vi "BCU诊断标定.vi"(8 "CAN端口":u16(ring), 9 "设备索引号":u16(ring), 10 "CAN卡类型":u32(ring)=21, 11 "Myindex":dbl=1.0) -> (3 "成功":bool)   [LabVIEW 2013] (continued)
              n483 = property class="Tree (严格)"(reference=w821, "Active Item Row Number"=9 ("活动项:行数"), "Disabled?"=w795, "Active Item Row Number"=1 ("活动项:行数"), "Disabled?"=w794, "Active Item Row Number"=0 ("活动项:行数"), "Disabled?"=w799, "Active Item Row Number"=3 ("活动项:行数"), "Disabled?"=w813, "Active Item Row Number"=4 ("活动项:行数"), "Disabled?"=w812, "Active Item Row Number"=5 ("活动项:行数"), "Disabled?"=w811, "Active Item Row Number"=6 ("活动项:行数"), "Disabled?"=w810, "Active Item Row Number"=7 ("活动项:行数"), "Disabled?"=w809, "Active Item Row Number"=8 ("活动项:行数"), "Disabled?"=w808, "Active Item Row Number"=11 ("活动项:行数"), "Disabled?"=w807, "Active Item Row Number"=12 ("活动项:行数"), "Disabled?"=w806, "Active Item Row Number"=13 ("活动项:行数"), "Disabled?"=w805, "Active Item Row Number"=2 ("活动项:行数"), "Disabled?"=w804, "Active Item Row Number"=10 ("活动项:行数"), "Disabled?"=w803, "Active Item Row Number"=14 ("活动项:行数"), "Disabled?"=w802) -> ()  [unwired: 1 in, 2 out]
            }
            frame #2 {
              w864 = 18
              # "一二三级故障"
              n484 = global read "功能码全局.vi" "主板故障阀值9"() -> (w870:bool[])
              n485 = Index Array(array=w870) -> (element #3=w869:bool, element #4=w866:bool, element #5=w863:bool, element #6=w868:bool, element #7=w865:bool, element #8=w862:bool)  [unwired: 8 in, 2 out]
              n486 = Not Or(1:w868, 2:w869) -> (0:w858:bool)
              n487 = Not Or(1:w865, 2:w866) -> (0:w856:bool)
              n488 = Not Or(1:w862, 2:w863) -> (0:w857:bool)
              n489 = for {
                N: w864 -> [_]
                tunnel: w859 -> [w890]
                tunnel: w858 -> [w886]
                tunnel: [w885] -> w867
                i -> [w888]
                n490 = Add(x=w888, y=15) -> (x+y=w889:i32)
                n491 = property class="Tree (严格)"(reference=w890, "Active Item Row Number"=w889, "Disabled?"=w886) -> (error out=w885:errorcluster)  [unwired: 1 in, 1 out]
              }
              n492 = for {
                N: w864 -> [_]
                tunnel: w859 -> [w884]
                tunnel: w856 -> [w880]
                tunnel: w867 -> [w879]
                tunnel: [w878] -> w861
                i -> [w882]
                n493 = Add(x=w882, y=33) -> (x+y=w883:i32)
                n494 = property class="Tree (严格)"(reference=w884, error in=w879, "Active Item Row Number"=w883, "Disabled?"=w880) -> (error out=w878:errorcluster)  [unwired: 1 out]
              }
              n495 = for {
                N: w864 -> [_]
                tunnel: w859 -> [w877]
                tunnel: w857 -> [w873]
                tunnel: w861 -> [w872]
                tunnel: [w871] -> w860
                i -> [w875]
                n496 = Add(x=w875, y=51) -> (x+y=w876:i32)
                n497 = property class="Tree (严格)"(reference=w877, error in=w872, "Active Item Row Number"=w876, "Disabled?"=w873) -> (error out=w871:errorcluster)  [unwired: 1 out]
              }
              n498 = call <vilib>:"Clear Errors.vi"("error in (no error)"=w860) -> ()  [unwired: 6 in, 1 out]
            }
          }
        }
        frame Enabled {
        }
      }
      n499 = disable-structure shown="禁用" {
        disable-tunnel: [w543 _] -> w542
        frame Disabled {
          n500 = control-ref of="从板选项"() -> (w544:refnum<vi>)
          n501 = stacked-sequence {
            tunnel: w544 -> [w547 w584 w626]
            tunnel: [w545 _ _] -> w543
            frame #0 {
              n502 = global read "功能码全局.vi" "15"() -> (w570:bool[])
              n503 = global read "功能码全局.vi" "16"() -> (w561:bool[])
              n504 = Index Array(array=w570) -> (element #1=w569:bool, element #2=w567:bool, element #3=w565:bool, element #4=w563:bool, element #5=w568:bool, element #6=w566:bool, element #7=w564:bool, element #8=w562:bool)  [unwired: 8 in]
              n505 = Index Array(array=w561) -> (element #5=w552:bool, element #6=w560:bool, element #7=w551:bool, element #8=w559:bool)  [unwired: 8 in, 4 out]
              n506 = Not Or(1:w559, 2:w560) -> (0:w549:bool)
              n507 = Not Or(1:w551, 2:w552) -> (0:w550:bool)
              n508 = Not Or(1:w568, 2:w569) -> (0:w555:bool)
              n509 = Not Or(1:w566, 2:w567) -> (0:w556:bool)
              n510 = Not Or(1:w564, 2:w565) -> (0:w557:bool)
              n511 = Not Or(1:w562, 2:w563) -> (0:w558:bool)
              n512 = Compound Arithmetic op=OR(w555, w556, w557, w558, w549) -> (w554:bool)
              "从板项目信息" <- w554
              n513 = property class="Tree (严格)"(reference=w547, "Active Item Row Number"=1 ("活动项:行数"), "Disabled?"=w554, "Active Item Row Number"=2 ("活动项:行数"), "Disabled?"=w555, "Active Item Row Number"=3 ("活动项:行数"), "Disabled?"=w556, "Active Item Row Number"=4 ("活动项:行数"), "Disabled?"=w557, "Active Item Row Number"=5 ("活动项:行数"), "Disabled?"=w558, "Active Item Row Number"=0 ("活动项:行数"), "Disabled?"=w550) -> (error out=w546:errorcluster)  [unwired: 1 in, 1 out]
              n514 = for {
                N: 8 -> [_]
                tunnel: w547 -> [w582]
                tunnel: w549 -> [w578]
                tunnel: w546 -> [w577]
                tunnel: [w576] -> w545
                i -> [w580]
                n515 = Add(x=w580, y=6) -> (x+y=w581:i32)
                n516 = property class="Tree (严格)"(reference=w582, error in=w577, "Active Item Row Number"=w581, "Disabled?"=w578) -> (error out=w576:errorcluster)  [unwired: 1 out]
              }
              n517 = call <vilib>:"Clear Errors.vi"("error in (no error)"=w545) -> ()  [unwired: 6 in, 1 out]
            }
            frame #1 {
              w595 = 8
              n518 = global read "功能码全局.vi" "18"() -> (w604:bool[])
              n519 = Index Array(array=w604) -> (element #1=w587:bool, element #2=w588:bool, element #3=w603:bool, element #4=w598:bool, element #5=w592:bool, element #6=w602:bool, element #7=w597:bool, element #8=w591:bool)  [unwired: 8 in]
              n520 = Not Or(1:w588, 2:w587) -> (0:w583:bool)
              n521 = property class="Tree (严格)"(reference=w584, "Active Item Row Number"=46 ("活动项:行数"), "Disabled?"=w583, "Active Item Row Number"=47 ("活动项:行数"), "Disabled?"=w583, "Active Item Row Number"=48 ("活动项:行数"), "Disabled?"=w583) -> ()  [unwired: 1 in, 2 out]
              n522 = Not Or(1:w591, 2:w592) -> (0:w590:bool)
              n523 = Not Or(1:w602, 2:w603) -> (0:w601:bool)
              n524 = Not Or(1:w597, 2:w598) -> (0:w596:bool)
              n525 = for {
                N: w595 -> [_]
                tunnel: w584 -> [w625]
                tunnel: w601 -> [w621]
                tunnel: "error out" -> [w620]
                tunnel: [w619] -> w599
                i -> [w623]
                n526 = Add(x=w623, y=14) -> (x+y=w624:i32)
                n527 = property class="Tree (严格)"(reference=w625, error in=w620, "Active Item Row Number"=w624, "Disabled?"=w621) -> (error out=w619:errorcluster)  [unwired: 1 out]
              }
              n528 = for {
                N: w595 -> [_]
                tunnel: w584 -> [w618]
                tunnel: w596 -> [w614]
                tunnel: w599 -> [w613]
                tunnel: [w612] -> w594
                i -> [w616]
                n529 = Add(x=w616, y=22) -> (x+y=w617:i32)
                n530 = property class="Tree (严格)"(reference=w618, error in=w613, "Active Item Row Number"=w617, "Disabled?"=w614) -> (error out=w612:errorcluster)  [unwired: 1 out]
              }
              n531 = for {
                N: w595 -> [_]
                tunnel: w584 -> [w611]
                tunnel: w590 -> [w607]
                tunnel: w594 -> [w606]
                tunnel: [w605] -> w593
                i -> [w609]
                n532 = Add(x=w609, y=30) -> (x+y=w610:i32)
                n533 = property class="Tree (严格)"(reference=w611, error in=w606, "Active Item Row Number"=w610, "Disabled?"=w607) -> (error out=w605:errorcluster)  [unwired: 1 out]
              }
              n534 = call <vilib>:"Clear Errors.vi"("error in (no error)"=w593) -> ()  [unwired: 6 in, 1 out]
            }
            frame #2 {
              n535 = global read "功能码全局.vi" "23"() -> (w650:bool[])
              n536 = global read "功能码全局.vi" "24"() -> (w648:bool[])
              n537 = Index Array(array=w650) -> (element #3=w649:bool, element #4=w646:bool, element #5=w644:bool, element #6=w642:bool, element #7=w640:bool, element #8=w638:bool)  [unwired: 8 in, 2 out]
              n538 = Index Array(array=w648) -> (element #3=w647:bool, element #4=w645:bool, element #5=w643:bool, element #6=w641:bool, element #7=w639:bool, element #8=w637:bool)  [unwired: 8 in, 2 out]
              n539 = Not Or(1:w647, 2:w649) -> (0:w636:bool)
              n540 = Not Or(1:w645, 2:w646) -> (0:w631:bool)
              n541 = Not Or(1:w643, 2:w644) -> (0:w632:bool)
              n542 = Not Or(1:w641, 2:w642) -> (0:w633:bool)
              n543 = Not Or(1:w639, 2:w640) -> (0:w635:bool)
              n544 = Not Or(1:w637, 2:w638) -> (0:w634:bool)
              n545 = Build Array(w636, w636, w635, w634, w633, w632, w631) -> (w629:bool[])
              n546 = And Array Elements(Boolean array=w629) -> (logical AND=w630:bool)
              n547 = Insert Into Array(array=w629, index=0 ("索引"), new element=w630) -> (w627:bool[])
              n548 = for {
                N: 8 -> [_]
                tunnel: w626 -> [w660]
                tunnel: w627 -> [w656] mode=indexing
                tunnel: errorcluster {"status"=FALSE, "code"=0, "source"=""} ("error out 2") -> [w655]
                tunnel: [w654] -> w652
                i -> [w658]
                n549 = Add(x=w658, y=38) -> (x+y=w659:i32)
                n550 = property class="Tree (严格)"(reference=w660, error in=w655, "Active Item Row Number"=w659, "Disabled?"=w656) -> (error out=w654:errorcluster)  [unwired: 1 out]
              }
              n551 = call <vilib>:"Clear Errors.vi"("error in (no error)"=w652) -> ()  [unwired: 6 in, 1 out]
            }
          }
        }
        frame Enabled {
        }
      }
    }
  }
  n552 = Obtain Queue(name (unnamed)=w46, element data type=w46, error in (no error)=w34) -> (queue out=w45:refnum<queue>, error out=w8:errorcluster)  [unwired: 2 in, 1 out]
  n553 = Number To Decimal String(number="Myindex") -> (decimal integer string=w2:string)  [unwired: 1 in]
  n554 = Obtain Queue(name (unnamed)=w2, element data type="读参数") -> (queue out=w39:refnum<queue>, error out=w38:errorcluster)  [unwired: 3 in, 1 out]
  n555 = call <vilib>:"Open Config Data.vi"("error in (no error)"=w8, "configuration file path"=path "D:/BlueWay/BMU从板号.ini") -> ("error out"=w6:errorcluster, "refnum"=w7:T19)  [unwired: 7 in, 1 out]
  n556 = call-poly <vilib>:"Read Key.vi"("section"=w11, "error in (no error)"=w6, "default value"="BNET0001", "key"=w11, "refnum"=w7) -> ("error out"=w12:errorcluster, "value"=w4:string, "refnum out"=w13:T19)  [unwired: 3 in, 1 out]
  n557 = disable-structure shown="启用" {
    disable-tunnel: w45 -> [w898 _]
    disable-tunnel: w8 -> [w897 _]
    disable-tunnel: w37 -> [w892 _]
    disable-tunnel: w34 -> [w891 _]
    frame Enabled {
      n558 = while {
        tunnel: w898 -> [w907]
        tunnel: w897 -> [w906]
        tunnel: [w905] -> w896
        tunnel: [w904] -> w895
        tunnel: w892 -> [_]
        tunnel: w891 -> [_]
        stop <- w903 stop-if-true
        n559 = event shown="[2] 前面板关闭？" {
          selector: _ -> [_ _ _ _ _ _ _ _ _ _ _ _ _ _ _ _ _ _ _ _ _ _ _ _ _ _ _ _ _ _ _ _ _ _ _ _ _ _ _ _ _ _ _ _ _ _ _ _ _ _ _ _ _]
          dyn-events: _ -> [_ _ _ _ _ _ _ _ _ _ _ _ _ _ _ _ _ _ _ _ _ _ _ _ _ _ _ _ _ _ _ _ _ _ _ _ _ _ _ _ _ _ _ _ _ _ _ _ _ _ _ _ _]
          timeout: 200 -> [_ _ _ _ _ _ _ _ _ _ _ _ _ _ _ _ _ _ _ _ _ _ _ _ _ _ _ _ _ _ _ _ _ _ _ _ _ _ _ _ _ _ _ _ _ _ _ _ _ _ _ _ _]
          tunnel: [w908 w911 w951 _ _ _ _ _ _ _ _ _ _ _ _ _ _ _ _ _ _ _ _ _ _ _ _ _ _ _ _ _ _ _ _ _ _ _ _ _ _ _ _ _ _ _ _ _ _ _ _ _ _] -> w902
          tunnel: w907 -> [w910 w914 w950 _ w991 w1002 w1013 w1024 w1035 w1046 w1057 w1068 w1079 w1090 w1101 w1112 w1128 w1651 w2063 w2088 w2116 w2219 w2292 w2305 w2315 w2361 _ _ w2411 w2478 w2545 w2612 w2679 w2746 w2813 w2881 w2949 w3016 w3083 w3153 w3164 w3203 w3243 w3283 w3323 w3361 w3421 w3456 w3492 w3525 w3595 w3628 w3661]
          tunnel: w906 -> [w909 w913 w949 _ w990 w1001 w1012 w1023 w1034 w1045 w1056 w1067 w1078 w1089 w1100 w1111 w1127 w1650 w2062 w2087 w2115 w2218 w2290 w2303 w2314 w2360 _ _ w2410 w2477 w2544 w2611 w2678 w2745 w2812 w2880 w2948 w3015 w3082 w3151 w3163 w3202 w3242 w3282 w3322 w3360 w3420 w3455 w3491 w3524 w3594 w3627 w3660]
          tunnel: [w910 w914 w950 _ w991 w1002 w1013 w1024 w1035 w1046 w1057 w1068 w1079 w1090 w1101 w1112 w1128 w1651 w2063 w2088 w2116 w2219 w2291 w2304 w2315 w2361 _ _ w2411 w2478 w2545 w2612 w2679 w2746 w2813 w2881 w2949 w3016 w3083 w3152 w3162 w3201 w3241 w3281 w3321 w3361 w3419 w3454 w3490 w3523 w3593 w3626 w3659] -> w905
          tunnel: [w909 w913 w949 _ w990 w1001 w1012 w1023 w1034 w1045 w1056 w1067 w1078 w1089 w1100 w1111 w1127 w1650 w2062 w2087 w2115 w2218 w2289 w2302 w2314 w2360 _ _ w2410 w2477 w2544 w2611 w2678 w2745 w2812 w2880 w2948 w3015 w3082 w3150 w3161 w3200 w3240 w3280 w3320 w3360 w3418 w3453 w3489 w3522 w3592 w3625 w3658] -> w904
          tunnel: [_ _ _ _ _ _ _ _ _ _ _ _ _ _ _ _ _ _ _ _ _ _ _ _ _ _ _ _ _ _ _ _ _ _ _ _ _ _ _ _ w3161 w3200 w3240 w3280 w3320 _ w3418 w3453 w3489 w3522 w3592 w3625 w3658] -> w901
          event Timeout {
            n560 = event-data() -> ()  [unwired: 3 out]
            n561 = local read "停止"() -> (w908:bool)
          }
          event "停止": Value Change {
            n562 = event-data() -> ("NewVal"=w912:bool)  [unwired: 5 out]
            n563 = stacked-sequence {
              tunnel: w912 -> [w931 _]
              tunnel: [w931 _] -> w911
              frame #0 {
                n564 = global read "配置文件全局.vi" "诊断标定读取地址"() -> (w915:path)
                n565 = call <vilib>:"Application Directory.vi"() -> ("Application Directory"=w925:path)
                n566 = property class="VI"("FP.State"=T24."Hidden" ("前面板窗口:状态")) -> (reference out=w927:refnum<vi>, error out=w926:errorcluster)  [unwired: 2 in]
                n567 = Build Path(base path=w925, name or relative path="config.ini" ("名称或相对路径")) -> (appended path=w923:path)
                n568 = call <vilib>:"Open Config Data.vi"("configuration file path"=w923) -> ("error out"=w920:errorcluster, "refnum"=w922:T19)  [unwired: 8 in, 1 out]
                n569 = local write "停止"(TRUE ("停止")) -> ()
                n570 = property class="VI"(reference=w927, error in=w926, "Front Panel.Open"=FALSE ("前面板窗口:打开")) -> ()  [unwired: 2 out]
                n571 = call-poly <vilib>:"Write Key.vi"("section"="总信息", "error in (no error)"=w920, "value"=w915, "key"="诊断标定读取地址" ("section"), "refnum"=w922) -> ("error out"=w919:errorcluster, "refnum out"=w918:T19)  [unwired: 4 in, 1 out]
                n572 = call <vilib>:"Close Config Data.vi"("error in (no error)"=w919, "refnum"=w918) -> ("error out"=w917:errorcluster)  [unwired: 8 in, 1 out]
                n573 = call <vilib>:"Clear Errors.vi"("error in (no error)"=w917) -> ()  [unwired: 6 in, 1 out]
              }
              frame #1 {
                n574 = disable-structure shown="禁用" {
                  frame Disabled {
                    n575 = local read "设备索引号"() -> (w937:u16)
                    n576 = local read "CAN卡类型"() -> (w938:u32)
                    n577 = local read "CAN端口"() -> (w936:u16)
                    n578 = Build Array(7) -> (w933:i32[])
                    n579 = call "transmit-8.6.vi"("can卡类型"=w938, "设备索引号"=w937, "CAN端口"=w936, "ID"=418398080, "SendType"=u8 0, "Data"=w933) -> ()  [unwired: 3 in, 11 out]
                  }
                  frame Enabled {
                    w945 = u8 0 items=["Normal", "Listen Only"] ("工作方式")
                    w944 = u8 1 items=["Dual Filter", "Single Filter"] ("滤波方式")
                    n580 = local read "设备索引号"() -> (w940:u16)
                    n581 = local read "CAN卡类型"() -> (w939:u32)
                    n582 = local read "CAN端口"() -> (w941:u16)
                    n583 = call "CAN_Init-8.6.vi"("CAN卡类型"=w939, "设备索引号"=w940, "CAN端口"=w941, "操作类型"=enum16{"初始化CAN", "关闭CAN"}."初始化CAN", "滤波方式"=w944, "Accept Code"=u32 0, "簇"=T23 {"打开CAN"=FALSE, "初始化CAN"=TRUE, "开始CAN"=TRUE, "重启"=FALSE, "关闭CAN"=FALSE}, "Mask Code"=u32 4294967295 ("Accept Code"), "工作方式"=w945, "是否滤波"=FALSE) -> ()  [unwired: 4 in, 6 out]
                  }
                }
              }
            }
          }
          event Panel Close? {
            n584 = event-data() -> ()  [unwired: 5 out]
            n585 = stacked-sequence {
              tunnel: [w964 _] -> w951
              frame #0 {
                w964 = TRUE ("前面板窗口:打开")
                n586 = global read "配置文件全局.vi" "诊断标定读取地址"() -> (w953:path)
                n587 = call <vilib>:"Application Directory.vi"() -> ("Application Directory"=w963:path)
                n588 = property class="VI"("FP.State"=T24."Hidden" ("前面板窗口:状态")) -> (reference out=w966:refnum<vi>, error out=w965:errorcluster)  [unwired: 2 in]
                n589 = Build Path(base path=w963, name or relative path="config.ini" ("名称或相对路径")) -> (appended path=w961:path)
                n590 = call <vilib>:"Open Config Data.vi"("configuration file path"=w961) -> ("error out"=w958:errorcluster, "refnum"=w960:T19)  [unwired: 8 in, 1 out]
                n591 = property class="VI"(reference=w966, error in=w965, "Front Panel.Open"=FALSE ("前面板窗口:打开")) -> ()  [unwired: 2 out]
                n592 = call-poly <vilib>:"Write Key.vi"("section"="总信息", "error in (no error)"=w958, "value"=w953, "key"="诊断标定读取地址" ("section"), "refnum"=w960) -> ("error out"=w957:errorcluster, "refnum out"=w956:T19)  [unwired: 4 in, 1 out]
                n593 = call <vilib>:"Close Config Data.vi"("error in (no error)"=w957, "refnum"=w956) -> ("error out"=w955:errorcluster)  [unwired: 8 in, 1 out]
                n594 = call <vilib>:"Clear Errors.vi"("error in (no error)"=w955) -> ()  [unwired: 6 in, 1 out]
                n595 = local write "强制终止读写标记"(TRUE ("强制终止读写标记")) -> ()
                n596 = local write "停止"(w964) -> ()
              }
              frame #1 {
                w972 = u8 0 items=["Normal", "Listen Only"] ("工作方式")
                w973 = u8 1 items=["Dual Filter", "Single Filter"] ("滤波方式")
                n597 = local read "设备索引号"() -> (w977:u16)
                n598 = local read "CAN卡类型"() -> (w978:u32)
                n599 = local read "CAN端口"() -> (w976:u16)
                n600 = call "CAN_Init-8.6.vi"("CAN卡类型"=w978, "设备索引号"=w977, "CAN端口"=w976, "操作类型"=enum16{"初始化CAN", "关闭CAN"}."初始化CAN", "滤波方式"=w973, "Accept Code"=u32 0, "簇"=T23 {"打开CAN"=FALSE, "初始化CAN"=TRUE, "开始CAN"=TRUE, "重启"=FALSE, "关闭CAN"=FALSE}, "Mask Code"=u32 4294967295 ("Accept Code"), "工作方式"=w972, "是否滤波"=FALSE) -> ()  [unwired: 4 in, 6 out]
              }
            }
            n601 = event-data("Discard?"=w951) -> ()  [unwired: 1 in, 1 out]
          }
          event "终止读写按钮": Value Change {
            n602 = event-data() -> ("NewVal"=w979:bool)  [unwired: 6 out]
            n603 = case shown="真" w979 {
              frame False {
              }
              frame True {
                n604 = local write "强制终止读写标记"(TRUE ("强制终止读写标记")) -> ()
              }
            }
          }
          event "1": Value Change {
            w988 = FALSE ("1")
            n605 = event-data() -> ()  [unwired: 7 out]
            n606 = local write "主板2"(T8."项目信息" ("主从板")) -> ()
            n607 = Not(x=w988) -> (.not. x?=w987:bool)
            n608 = local write "1"(w987) -> ()
            n609 = local write "1 2"(w988) -> ()
            n610 = local write "1 3"(w988) -> ()
            n611 = local write "1 4"(w988) -> ()
            n612 = local write "1 5"(w988) -> ()
            n613 = local write "1 11"(w988) -> ()
            n614 = global read "功能码全局.vi" "主板监控2"() -> (w986:bool[])
            n615 = Index Array(array=w986, index=6 ("索引")) -> (element=w981:bool)
            n616 = Select(t=0, s=w981, f=1) -> (s? t:f=w982:i32)
            n617 = property on="项目信息" class="Tbl (严格)"("Disabled"=w982) -> ()  [unwired: 2 in, 2 out]
            n618 = property on="电池实际容量(A)" class="DigNum (严格)"("Disabled"=w982) -> ()  [unwired: 2 in, 2 out]
            n619 = property on="使用者" class="DigNum (严格)"("Disabled"=w982) -> ()  [unwired: 2 in, 2 out]
            n620 = property on="SOH(%)" class="DigNum (严格)"("Disabled"=w982) -> ()  [unwired: 2 in, 2 out]
            n621 = property on="电池额定容量(A)" class="DigNum (严格)"("Disabled"=w982) -> ()  [unwired: 2 in, 2 out]
            n622 = property on="SOC(%)" class="DigNum (严格)"("Disabled"=w982) -> ()  [unwired: 2 in, 2 out]
            n623 = property on="项目信息2" class="Clust (严格)"("DisabledEnum"=w982) -> ()  [unwired: 2 in, 2 out]
            n624 = property on="系统时钟" class="Str"("Disabled"=w982) -> ()  [unwired: 2 in, 2 out]
            n625 = property on="配置文件版本" class="Str"("Disabled"=w982) -> ()  [unwired: 2 in, 2 out]
            n626 = property on="车架(牌)号" class="Str"("Disabled"=w982) -> ()  [unwired: 2 in, 2 out]
            n627 = property on="产品编号" class="Str"("Disabled"=w982) -> ()  [unwired: 2 in, 2 out]
          }
          event "1 2": Value Change {
            w999 = FALSE ("1")
            n628 = event-data() -> ()  [unwired: 7 out]
            n629 = local write "主板2"(T8."一级故障阀值" ("主从板")) -> ()
            n630 = Not(x=w999) -> (.not. x?=w998:bool)
            n631 = local write "1"(w999) -> ()
            n632 = local write "1 2"(w998) -> ()
            n633 = local write "1 3"(w999) -> ()
            n634 = local write "1 4"(w999) -> ()
            n635 = local write "1 5"(w999) -> ()
            n636 = local write "1 11"(w999) -> ()
            n637 = global read "功能码全局.vi" "主板监控2"() -> (w997:bool[])
            n638 = Index Array(array=w997, index=6 ("索引")) -> (element=w992:bool)
            n639 = Select(t=0, s=w992, f=1) -> (s? t:f=w995:i32)
            n640 = property on="一级故障" class="Clust (严格)"("DisabledEnum"=w995) -> ()  [unwired: 2 in, 2 out]
          }
          event "1 3": Value Change {
            w1010 = FALSE ("1")
            n641 = event-data() -> ()  [unwired: 7 out]
            n642 = local write "主板2"(T8."二级故障阀值" ("主从板")) -> ()
            n643 = Not(x=w1010) -> (.not. x?=w1009:bool)
            n644 = local write "1"(w1010) -> ()
            n645 = local write "1 2"(w1010) -> ()
            n646 = local write "1 3"(w1009) -> ()
            n647 = local write "1 4"(w1010) -> ()
            n648 = local write "1 5"(w1010) -> ()
            n649 = local write "1 11"(w1010) -> ()
            n650 = global read "功能码全局.vi" "主板监控2"() -> (w1008:bool[])
            n651 = Index Array(array=w1008, index=6 ("索引")) -> (element=w1004:bool)
            n652 = Select(t=0, s=w1004, f=1) -> (s? t:f=w1003:i32)
            n653 = property on="一级故障 2" class="Clust (严格)"("DisabledEnum"=w1003) -> ()  [unwired: 2 in, 2 out]
          }
          event "1 4": Value Change {
            w1021 = FALSE ("1")
            n654 = event-data() -> ()  [unwired: 7 out]
            n655 = local write "主板2"(T8."三级故障阀值" ("主从板")) -> ()
            n656 = Not(x=w1021) -> (.not. x?=w1020:bool)
            n657 = local write "1"(w1021) -> ()
            n658 = local write "1 2"(w1021) -> ()
            n659 = local write "1 3"(w1021) -> ()
            n660 = local write "1 4"(w1020) -> ()
            n661 = local write "1 5"(w1021) -> ()
            n662 = local write "1 11"(w1021) -> ()
            n663 = global read "功能码全局.vi" "主板监控2"() -> (w1019:bool[])
            n664 = Index Array(array=w1019, index=6 ("索引")) -> (element=w1014:bool)
            n665 = Select(t=0, s=w1014, f=1) -> (s? t:f=w1017:i32)
            n666 = property on="一级故障 3" class="Clust (严格)"("DisabledEnum"=w1017) -> ()  [unwired: 2 in, 2 out]
          }
          event "1 5": Value Change {
            w1032 = FALSE ("1")
            n667 = event-data() -> ()  [unwired: 7 out]
            n668 = local write "主板2"(T8."控制参数" ("主从板")) -> ()
            n669 = Not(x=w1032) -> (.not. x?=w1031:bool)
            n670 = local write "1"(w1032) -> ()
            n671 = local write "1 2"(w1032) -> ()
            n672 = local write "1 3"(w1032) -> ()
            n673 = local write "1 4"(w1032) -> ()
            n674 = local write "1 5"(w1031) -> ()
            n675 = local write "1 11"(w1032) -> ()
            n676 = global read "功能码全局.vi" "主板监控2"() -> (w1028:bool[])
            n677 = Index Array(array=w1028, index=6 ("索引")) -> (element=w1026:bool)
            n678 = Select(t=0, s=w1026, f=1) -> (s? t:f=w1025:i32)
            n679 = property on="风机开启温度" class="DigNum (严格)"("Disabled"=w1025) -> ()  [unwired: 2 in, 2 out]
            n680 = property on="风机关闭温度" class="DigNum (严格)"("Disabled"=w1025) -> ()  [unwired: 2 in, 2 out]
            n681 = property on="加热开启温度" class="DigNum (严格)"("Disabled"=w1025) -> ()  [unwired: 2 in, 2 out]
            n682 = property on="加热关闭温度" class="DigNum (严格)"("Disabled"=w1025) -> ()  [unwired: 2 in, 2 out]
            n683 = property on="风机开启温差" class="DigNum (严格)"("Disabled"=w1025) -> ()  [unwired: 2 in, 2 out]
            n684 = property on="风机关闭温差" class="DigNum (严格)"("Disabled"=w1025) -> ()  [unwired: 2 in, 2 out]
            n685 = property on="加热控制参数" class="Clust (严格)"("DisabledEnum"=w1025) -> ()  [unwired: 2 in, 2 out]
            n686 = property on="最大允许总电压" class="DigNum (严格)"("Disabled"=w1025) -> ()  [unwired: 2 in, 2 out]
            n687 = property on="最大允许充电温度" class="DigNum (严格)"("Disabled"=w1025) -> ()  [unwired: 2 in, 2 out]
            n688 = property on="最小允许充电温度" class="DigNum (严格)"("Disabled"=w1025) -> ()  [unwired: 2 in, 2 out]
            n689 = property on="电流步长" class="DigNum (严格)"("Disabled"=w1025) -> ()  [unwired: 2 in, 2 out]
            n690 = property on="最大允许单体电压" class="DigNum (严格)"("Disabled"=w1025) -> ()  [unwired: 2 in, 2 out]
            n691 = property on="最小允许单体电压" class="DigNum (严格)"("Disabled"=w1025) -> ()  [unwired: 2 in, 2 out]
            n692 = property on="最大允许充电电流" class="DigNum (严格)"("Disabled"=w1025) -> ()  [unwired: 2 in, 2 out]
            n693 = property on="最小允许充电电流" class="DigNum (严格)"("Disabled"=w1025) -> ()  [unwired: 2 in, 2 out]
          }
          event "1 11": Value Change {
            w1043 = FALSE ("1")
            n694 = event-data() -> ()  [unwired: 7 out]
            n695 = local write "主板2"(T8."电池信息" ("主从板")) -> ()
            n696 = Not(x=w1043) -> (.not. x?=w1042:bool)
            n697 = local write "1"(w1043) -> ()
            n698 = local write "1 2"(w1043) -> ()
            n699 = local write "1 3"(w1043) -> ()
            n700 = local write "1 4"(w1043) -> ()
            n701 = local write "1 5"(w1043) -> ()
            n702 = local write "1 11"(w1042) -> ()
            n703 = global read "功能码全局.vi" "主板监控2"() -> (w1038:bool[])
            n704 = Index Array(array=w1038, index=6 ("索引")) -> (element=w1036:bool)
            n705 = Select(t=0, s=w1036, f=1) -> (s? t:f=w1039:i32)
            n706 = property on="电池串联" class="DigNum (严格)"("Disabled"=w1039) -> ()  [unwired: 2 in, 2 out]
            n707 = property on="电池并联" class="DigNum (严格)"("Disabled"=w1039) -> ()  [unwired: 2 in, 2 out]
            n708 = property on="电池包额定容量" class="DigNum (严格)"("Disabled"=w1039) -> ()  [unwired: 2 in, 2 out]
            n709 = property on="电池包额定能量(kWh)" class="DigNum (严格)"("Disabled"=w1039) -> ()  [unwired: 2 in, 2 out]
            n710 = property on="电池包额定总电压" class="DigNum (严格)"("Disabled"=w1039) -> ()  [unwired: 2 in, 2 out]
            n711 = property on="实际容量" class="DigNum (严格)"("Disabled"=w1039) -> ()  [unwired: 2 in, 2 out]
            n712 = property on="电池包组号" class="Str"("Disabled"=w1039) -> ()  [unwired: 2 in, 2 out]
            n713 = property on="电池生产日期" class="Str"("Disabled"=w1039) -> ()  [unwired: 2 in, 2 out]
            n714 = property on="电池厂家" class="Str"("Disabled"=w1039) -> ()  [unwired: 2 in, 2 out]
            n715 = property on="电池类型" class="Str"("Disabled"=w1039) -> ()  [unwired: 2 in, 2 out]
            n716 = property on="累计充电总安时" class="DigNum (严格)"("Disabled"=w1039) -> ()  [unwired: 2 in, 2 out]
            n717 = property on="累计放电总安时" class="DigNum (严格)"("Disabled"=w1039) -> ()  [unwired: 2 in, 2 out]
            n718 = property on="电池放空次数" class="DigNum (严格)"("Disabled"=w1039) -> ()  [unwired: 2 in, 2 out]
            n719 = property on="电池充满次数" class="DigNum (严格)"("Disabled"=w1039) -> ()  [unwired: 2 in, 2 out]
            n720 = property on="电池充电次数" class="DigNum (严格)"("Disabled"=w1039) -> ()  [unwired: 2 in, 2 out]
            n721 = property on="电池信息" class="Clust (严格)"("DisabledEnum"=w1039) -> ()  [unwired: 2 in, 2 out]
          }
          event "1 6": Value Change {
            w1054 = FALSE ("1 6")
            n722 = event-data() -> ()  [unwired: 7 out]
            n723 = local write "等级 2"(T21."从板信息" ("等级 2")) -> ()
            n724 = global read "功能码全局.vi" "主板监控2"() -> (w1049:bool[])
            n725 = Not(x=w1054) -> (.not. x?=w1053:bool)
            n726 = local write "1 6"(w1053) -> ()
            n727 = local write "1 7"(w1054) -> ()
            n728 = local write "1 8"(w1054) -> ()
            n729 = local write "1 9"(w1054) -> ()
            n730 = local write "1 10"(w1054) -> ()
            n731 = Index Array(array=w1049, index=6 ("索引")) -> (element=w1047:bool)
            n732 = Select(t=0, s=w1047, f=1) -> (s? t:f=w1050:i32)
            n733 = property on="项目信息 2" class="Tbl (严格)"("Disabled"=w1050) -> ()  [unwired: 2 in, 2 out]
            n734 = property on="加热控制参数" class="Clust (严格)"("Disabled"=w1050) -> ()  [unwired: 2 in, 2 out]
          }
          event "1 7": Value Change {
            w1065 = FALSE ("1 6")
            n735 = event-data() -> ()  [unwired: 7 out]
            n736 = global read "功能码全局.vi" "主板监控2"() -> (w1063:bool[])
            n737 = Index Array(array=w1063, index=6 ("索引")) -> (element=w1058:bool)
            n738 = local write "等级 2"(T21."一级故障阀值" ("等级 2")) -> ()
            n739 = Select(t=0, s=w1058, f=1) -> (s? t:f=w1059:i32)
            n740 = property on="一级故障 6" class="Clust (严格)"("DisabledEnum"=w1059) -> ()  [unwired: 2 in, 2 out]
            n741 = Not(x=w1065) -> (.not. x?=w1064:bool)
            n742 = local write "1 6"(w1065) -> ()
            n743 = local write "1 7"(w1064) -> ()
            n744 = local write "1 8"(w1065) -> ()
            n745 = local write "1 9"(w1065) -> ()
            n746 = local write "1 10"(w1065) -> ()
          }
          event "1 8": Value Change {
            w1076 = FALSE ("1 6")
            n747 = event-data() -> ()  [unwired: 7 out]
            n748 = global read "功能码全局.vi" "主板监控2"() -> (w1074:bool[])
            n749 = Index Array(array=w1074, index=6 ("索引")) -> (element=w1069:bool)
            n750 = local write "等级 2"(T21."二级故障阀值" ("等级 2")) -> ()
            n751 = Select(t=0, s=w1069, f=1) -> (s? t:f=w1070:i32)
            n752 = Not(x=w1076) -> (.not. x?=w1075:bool)
            n753 = property on="一级故障 7" class="Clust (严格)"("DisabledEnum"=w1070) -> ()  [unwired: 2 in, 2 out]
            n754 = local write "1 6"(w1076) -> ()
            n755 = local write "1 7"(w1076) -> ()
            n756 = local write "1 8"(w1075) -> ()
            n757 = local write "1 9"(w1076) -> ()
            n758 = local write "1 10"(w1076) -> ()
          }
          event "1 9": Value Change {
            w1087 = FALSE ("1 6")
            n759 = event-data() -> ()  [unwired: 7 out]
            n760 = global read "功能码全局.vi" "主板监控2"() -> (w1085:bool[])
            n761 = Index Array(array=w1085, index=6 ("索引")) -> (element=w1080:bool)
            n762 = Select(t=0, s=w1080, f=1) -> (s? t:f=w1081:i32)
            n763 = local write "等级 2"(T21."三级故障阀值" ("等级 2")) -> ()
            n764 = property on="一级故障 8" class="Clust (严格)"("DisabledEnum"=w1081) -> ()  [unwired: 2 in, 2 out]
            n765 = Not(x=w1087) -> (.not. x?=w1086:bool)
            n766 = local write "1 6"(w1087) -> ()
            n767 = local write "1 7"(w1087) -> ()
            n768 = local write "1 8"(w1087) -> ()
            n769 = local write "1 9"(w1086) -> ()
            n770 = local write "1 10"(w1087) -> ()
          }
          event "1 10": Value Change {
            w1098 = FALSE ("1 6")
            n771 = event-data() -> ()  [unwired: 7 out]
            n772 = global read "功能码全局.vi" "主板监控2"() -> (w1096:bool[])
            n773 = Index Array(array=w1096, index=6 ("索引")) -> (element=w1091:bool)
            n774 = Select(t=0, s=w1091, f=1) -> (s? t:f=w1092:i32)
            n775 = local write "等级 2"(T21."快换参数" ("等级 2")) -> ()
            n776 = property on="电池组信息" class="Clust (严格)"("Disabled"=w1092) -> ()  [unwired: 2 in, 2 out]
            n777 = Not(x=w1098) -> (.not. x?=w1097:bool)
            n778 = local write "1 6"(w1098) -> ()
            n779 = local write "1 7"(w1098) -> ()
            n780 = local write "1 8"(w1098) -> ()
            n781 = local write "1 9"(w1098) -> ()
            n782 = local write "1 10"(w1097) -> ()
          }
          event "1 12": Value Change {
            w1103 = FALSE ("1 6")
            n783 = event-data() -> ()  [unwired: 7 out]
            n784 = global read "功能码全局.vi" "主板监控2"() -> (w1110:bool[])
            n785 = Index Array(array=w1110, index=6 ("索引")) -> (element=w1106:bool)
            n786 = Select(t=0, s=w1106, f=1) -> (s? t:f=w1102:i32)
            n787 = local write "等级 2"(T14."均衡参数" ("等级 2")) -> ()
            n788 = property on="均衡参数" class="Clust (严格)"("DisabledEnum"=w1102) -> ()  [unwired: 2 in, 2 out]
            n789 = Not(x=w1103) -> (.not. x?=w1104:bool)
            n790 = local write "1 12"(w1104) -> ()
            n791 = local write "1 6"(w1103) -> ()
            n792 = local write "1 7"(w1103) -> ()
            n793 = local write "1 8"(w1103) -> ()
            n794 = local write "1 9"(w1103) -> ()
            n795 = local write "1 10"(w1103) -> ()
          }
          event "主板选项": Mouse Down {
            n796 = event-data() -> ("CtlRef"=w1126:refnum<vi>)  [unwired: 8 out]
            n797 = global read "功能码全局.vi" "主板监控2"() -> (w1115:bool[])
            n798 = property class="Tree (严格)"(reference=w1126) -> ("Value"=w1118:string)  [unwired: 1 in, 2 out]
            n799 = Index Array(array=w1115, index=6 ("索引")) -> (element=w1113:bool)
            n800 = case shown="\"温度个数\"" w1118 {
              tunnel: [T8."项目信息" ("主从板") T8."项目信息" ("主从板") T8."项目信息" ("主从板") T8."项目信息" ("主从板") T8."项目信息" ("主从板") T8."项目信息" ("主从板") T8."项目信息" ("主从板") T8."项目信息" ("主从板") T8."项目信息" ("主从板") T8."项目信息" ("主从板") T8."项目信息" ("主从板") T8."项目信息" ("主从板") T8."项目信息" ("主从板") T8."项目信息" ("主从板") T8."项目信息" ("主从板") T8."二级故障阀值" ("主从板") T8."三级故障阀值" ("主从板") T8."一级故障阀值" ("主从板") T8."控制参数" ("主从板") T8."控制参数" ("主从板") T8."电池信息" ("主从板") T8."电池信息" ("主从板") T8."电池信息" ("主从板") T8."电池信息" ("主从板") T8."电池信息" ("主从板") T8."项目信息" ("主从板")] -> w1125
              tunnel: [w1136 w1143 w1158 w1175 w1215 w1249 w1296 w1334 w1384 w1419 w1433 w1448 w1463 w1478 w1492 w1505 w1519 w1532 w1546 w1560 w1573 w1587 w1601 w1615 w1629 w1633] -> w1124
              tunnel: [w1137 w1144 w1159 w1176 w1216 w1250 w1297 w1335 w1385 w1420 w1434 w1449 w1464 w1479 w1493 w1505 w1519 w1531 w1546 w1560 w1573 w1587 w1601 w1615 w1629 w1634] -> w1123
              tunnel: [w1137 w1144 w1159 w1176 w1216 w1250 w1297 w1335 w1385 w1420 w1434 w1449 w1464 w1479 w1493 w1506 w1519 w1532 w1546 w1560 w1573 w1587 w1601 w1615 w1629 w1634] -> w1122
              tunnel: [w1137 w1144 w1159 w1176 w1216 w1250 w1297 w1335 w1385 w1420 w1434 w1449 w1464 w1479 w1493 w1505 w1518 w1532 w1546 w1560 w1573 w1587 w1601 w1615 w1629 w1634] -> w1121
              tunnel: [w1137 w1144 w1159 w1176 w1216 w1250 w1297 w1335 w1385 w1420 w1434 w1449 w1464 w1479 w1493 w1505 w1519 w1532 w1545 w1559 w1573 w1587 w1601 w1615 w1629 w1634] -> w1120
              tunnel: [w1137 w1144 w1159 w1176 w1216 w1250 w1297 w1335 w1385 w1420 w1434 w1449 w1464 w1479 w1493 w1505 w1519 w1532 w1546 w1560 w1572 w1586 w1600 w1614 w1628 w1634] -> w1119
              tunnel: [w1129 FALSE w1154 w1167 w1207 w1240 w1287 w1326 w1377 w1414 w1428 w1442 w1456 w1471 w1487 w1501 w1514 w1527 w1541 w1554 w1568 w1581 w1595 w1609 w1623 FALSE] -> w1117
              tunnel: [w1129 TRUE w1151 w1166 w1206 w1241 w1288 w1325 w1376 w1413 w1427 w1441 w1457 w1472 w1486 w1500 w1513 w1526 w1540 w1553 w1567 w1580 w1594 w1608 w1622 FALSE] -> w1116
              tunnel: w1113 -> [w1134 _ w1148 w1163 w1202 w1237 w1284 w1322 w1374 w1410 w1424 w1438 w1453 w1468 w1483 w1497 w1510 w1523 w1537 w1550 w1564 w1577 w1591 w1605 w1619 _]
              frame "项目信息" {
                w1137 = FALSE
                n801 = Select(t=0, s=w1134, f=1) -> (s? t:f=w1132:i32)
                n802 = property on="项目信息" class="Tbl (严格)"("Disabled"=w1132) -> ()  [unwired: 2 in, 2 out]
                n803 = property on="电池实际容量(A)" class="DigNum (严格)"("Disabled"=w1132) -> ()  [unwired: 2 in, 2 out]
                n804 = property on="使用者" class="DigNum (严格)"("Disabled"=w1132) -> ()  [unwired: 2 in, 2 out]
                n805 = property on="SOH(%)" class="DigNum (严格)"("Disabled"=w1132) -> ()  [unwired: 2 in, 2 out]
                n806 = property on="从板个数" class="DigNum (严格)"("NumText.BGColor"=u32 6618880) -> ()  [unwired: 2 in, 2 out]
                n807 = property on="电池额定容量(A)" class="DigNum (严格)"("Disabled"=w1132) -> ()  [unwired: 2 in, 2 out]
                n808 = property on="SOC(%)" class="DigNum (严格)"("Disabled"=w1132) -> ()  [unwired: 2 in, 2 out]
                n809 = property on="项目信息2" class="Clust (严格)"("DisabledEnum"=w1132) -> ()  [unwired: 2 in, 2 out]
                n810 = property on="系统时钟" class="Str"("Disabled"=w1132) -> ()  [unwired: 2 in, 2 out]
                n811 = property on="配置文件版本" class="Str"("Disabled"=w1132) -> ()  [unwired: 2 in, 2 out]
                n812 = property on="车架(牌)号" class="Str"("Disabled"=w1132) -> ()  [unwired: 2 in, 2 out]
                n813 = property on="产品编号" class="Str"("Disabled"=w1132) -> ()  [unwired: 2 in, 2 out]
                n814 = local read "项目信息结果"() -> (w1130:bool)
                n815 = Not(x=w1130) -> (.not. x?=w1129:bool)
                n816 = Not(x=w1137) -> (.not. x?=w1136:bool)
              }
              frame "校正时钟" {
                w1140 = 2
                w1144 = FALSE
                n817 = property on="从板个数" class="DigNum (严格)"("NumText.BGColor"=u32 13816530) -> ()  [unwired: 2 in, 2 out]
                n818 = property on="项目信息" class="Tbl (严格)"("Disabled"=w1140) -> ()  [unwired: 2 in, 2 out]
                n819 = property on="电池实际容量(A)" class="DigNum (严格)"("Disabled"=w1140) -> ()  [unwired: 2 in, 2 out]
                n820 = property on="使用者" class="DigNum (严格)"("Disabled"=w1140) -> ()  [unwired: 2 in, 2 out]
                n821 = property on="SOH(%)" class="DigNum (严格)"("Disabled"=w1140) -> ()  [unwired: 2 in, 2 out]
                n822 = property on="电池额定容量(A)" class="DigNum (严格)"("Disabled"=w1140) -> ()  [unwired: 2 in, 2 out]
                n823 = property on="SOC(%)" class="DigNum (严格)"("Disabled"=w1140) -> ()  [unwired: 2 in, 2 out]
                n824 = property on="系统时钟" class="Str"("Disabled"=w1140) -> ()  [unwired: 2 in, 2 out]
                n825 = property on="配置文件版本" class="Str"("Disabled"=w1140) -> ()  [unwired: 2 in, 2 out]
                n826 = property on="车架(牌)号" class="Str"("Disabled"=w1140) -> ()  [unwired: 2 in, 2 out]
                n827 = property on="项目信息2" class="Clust (严格)"("DisabledEnum"=w1140) -> ()  [unwired: 2 in, 2 out]
                n828 = property on="产品编号" class="Str"("Disabled"=w1140) -> ()  [unwired: 2 in, 2 out]
                n829 = Not(x=w1144) -> (.not. x?=w1143:bool)
              }
              frame "产品编号" {
                w1157 = 2
                w1159 = FALSE
                n830 = property on="项目信息" class="Tbl (严格)"("Disabled"=w1157) -> ()  [unwired: 2 in, 2 out]
                n831 = property on="电池实际容量(A)" class="DigNum (严格)"("Disabled"=w1157) -> ()  [unwired: 2 in, 2 out]
                n832 = property on="使用者" class="DigNum (严格)"("Disabled"=w1157) -> ()  [unwired: 2 in, 2 out]
                n833 = Select(t=0, s=w1148, f=1) -> (s? t:f=w1147:i32)
                n834 = property on="SOH(%)" class="DigNum (严格)"("Disabled"=w1157) -> ()  [unwired: 2 in, 2 out]
                n835 = property on="电池额定容量(A)" class="DigNum (严格)"("Disabled"=w1157) -> ()  [unwired: 2 in, 2 out]
                n836 = property on="SOC(%)" class="DigNum (严格)"("Disabled"=w1157) -> ()  [unwired: 2 in, 2 out]
                n837 = property on="产品编号" class="Str"("Disabled"=w1147) -> ()  [unwired: 2 in, 2 out]
                n838 = property on="项目信息2" class="Clust (严格)"("DisabledEnum"=w1147) -> ()  [unwired: 2 in, 2 out]
                n839 = property on="系统时钟" class="Str"("Disabled"=w1157) -> ()  [unwired: 2 in, 2 out]
                n840 = property on="配置文件版本" class="Str"("Disabled"=w1157) -> ()  [unwired: 2 in, 2 out]
                n841 = property on="车架(牌)号" class="Str"("Disabled"=w1157) -> ()  [unwired: 2 in, 2 out]
                n842 = property on="从板个数" class="DigNum (严格)"("NumText.BGColor"=u32 13816530) -> ()  [unwired: 2 in, 2 out]
                n843 = global read "功能码全局.vi" "主板项目信息5"() -> (w1155:bool[])
                n844 = global read "功能码全局.vi" "主板项目信息6"() -> (w1152:bool[])
                n845 = Index Array(array=w1155, index=0 ("索引")) -> (element=w1154:bool)
                n846 = Index Array(array=w1152, index=1 ("索引")) -> (element=w1151:bool)
                n847 = Not(x=w1159) -> (.not. x?=w1158:bool)
              }
              frame "电压个数" {
                w1174 = 2
                w1176 = FALSE
                n848 = local read "从板个数"() -> (w1173:dbl)
                n849 = property on="从板个数" class="DigNum (严格)"("NumText.BGColor"=u32 6618880) -> ()  [unwired: 2 in, 2 out]
                n850 = property on="电池实际容量(A)" class="DigNum (严格)"("Disabled"=w1174) -> ()  [unwired: 2 in, 2 out]
                n851 = property on="使用者" class="DigNum (严格)"("Disabled"=w1174) -> ()  [unwired: 2 in, 2 out]
                n852 = property on="SOH(%)" class="DigNum (严格)"("Disabled"=w1174) -> ()  [unwired: 2 in, 2 out]
                n853 = property on="电池额定容量(A)" class="DigNum (严格)"("Disabled"=w1174) -> ()  [unwired: 2 in, 2 out]
                n854 = property on="SOC(%)" class="DigNum (严格)"("Disabled"=w1174) -> ()  [unwired: 2 in, 2 out]
                n855 = property on="系统时钟" class="Str"("Disabled"=w1174) -> ()  [unwired: 2 in, 2 out]
                n856 = property on="配置文件版本" class="Str"("Disabled"=w1174) -> ()  [unwired: 2 in, 2 out]
                n857 = property on="车架(牌)号" class="Str"("Disabled"=w1174) -> ()  [unwired: 2 in, 2 out]
                n858 = property on="产品编号" class="Str"("Disabled"=w1174) -> ()  [unwired: 2 in, 2 out]
                n859 = Select(t=0, s=w1163, f=1) -> (s? t:f=w1162:i32)
                n860 = control-ref of="项目信息"() -> (w1172:refnum<vi>)
                n861 = stacked-sequence {
                  tunnel: w1173 -> [_ w1183 w1193]
                  tunnel: w1172 -> [w1178 w1182 w1194]
                  frame #0 {
                    w1179 = 0
                    n862 = Bundle(w1179, w1179) -> (w1181:cluster{i32, i32})  [unwired: 1 out]
                    n863 = property class="Tbl (严格)"(reference=w1178, "Index Values"=w1181) -> (error out=w1180:errorcluster)  [unwired: 1 in, 1 out]
                    n864 = call <vilib>:"Clear Errors.vi"("error in (no error)"=w1180) -> ()  [unwired: 7 out]
                  }
                  frame #1 {
                    n865 = for {
                      N: 10 -> [_]
                      tunnel: w1182 -> [w1192]
                      tunnel: w1183 -> [w1187]
                      i -> [w1186]
                      n866 = Compound Arithmetic op=ADD(0.0 ("值"), w1187, w1186) -> (w1189:dbl)
                      n867 = Bundle(w1189, 0) -> (w1191:cluster{dbl, i32})  [unwired: 1 out]
                      n868 = property class="Tbl (严格)"(reference=w1192, "Active Cell"=w1191, "Cell BG Color"=u32 16448250) -> ()  [unwired: 1 in, 2 out]
                    }
                  }
                  frame #2 {
                    n869 = for {
                      N: w1193 -> [_]
                      tunnel: w1194 -> [w1195]
                      i -> [w1196]
                      n870 = Bundle(w1196, 0) -> (w1200:cluster{i32, i32})  [unwired: 1 out]
                      n871 = property class="Tbl (严格)"(reference=w1195, "Active Cell"=w1200, "Cell BG Color"=u32 6618880) -> (error out=w1197:errorcluster)  [unwired: 1 in, 1 out]
                      n872 = call <vilib>:"Clear Errors.vi"("error in (no error)"=w1197) -> ()  [unwired: 7 out]
                    }
                  }
                }
                n873 = property on="项目信息" class="Tbl (严格)"("Disabled"=w1162) -> ()  [unwired: 2 in, 2 out]
                n874 = global read "功能码全局.vi" "主板项目信息5"() -> (w1170:bool[])
                n875 = global read "功能码全局.vi" "主板项目信息6"() -> (w1168:bool[])
                n876 = Index Array(array=w1170, index=1 ("索引")) -> (element=w1167:bool)
                n877 = Index Array(array=w1168, index=2 ("索引")) -> (element=w1166:bool)
                n878 = Not(x=w1176) -> (.not. x?=w1175:bool)
              }
              frame "通道电压数" {
                w1214 = 2
                w1216 = FALSE
                n879 = property on="从板个数" class="DigNum (严格)"("NumText.BGColor"=u32 13816530) -> ()  [unwired: 2 in, 2 out]
                n880 = property on="电池实际容量(A)" class="DigNum (严格)"("Disabled"=w1214) -> ()  [unwired: 2 in, 2 out]
                n881 = property on="使用者" class="DigNum (严格)"("Disabled"=w1214) -> ()  [unwired: 2 in, 2 out]
                n882 = property on="SOH(%)" class="DigNum (严格)"("Disabled"=w1214) -> ()  [unwired: 2 in, 2 out]
                n883 = property on="电池额定容量(A)" class="DigNum (严格)"("Disabled"=w1214) -> ()  [unwired: 2 in, 2 out]
                n884 = property on="SOC(%)" class="DigNum (严格)"("Disabled"=w1214) -> ()  [unwired: 2 in, 2 out]
                n885 = local read "从板个数"() -> (w1212:dbl)
                n886 = property on="系统时钟" class="Str"("Disabled"=w1214) -> ()  [unwired: 2 in, 2 out]
                n887 = property on="配置文件版本" class="Str"("Disabled"=w1214) -> ()  [unwired: 2 in, 2 out]
                n888 = property on="车架(牌)号" class="Str"("Disabled"=w1214) -> ()  [unwired: 2 in, 2 out]
                n889 = property on="产品编号" class="Str"("Disabled"=w1214) -> ()  [unwired: 2 in, 2 out]
                n890 = control-ref of="项目信息"() -> (w1213:refnum<vi>)
                n891 = stacked-sequence {
                  tunnel: w1213 -> [w1223 w1226]
                  tunnel: w1212 -> [w1222 w1225]
                  frame #0 {
                    n892 = Compound Arithmetic op=ADD(1.0 ("值"), w1222) -> (w1219:dbl)
                    n893 = Bundle(w1219, 0) -> (w1221:cluster{dbl, i32})  [unwired: 1 out]
                    n894 = property class="Tbl (严格)"(reference=w1223, "Index Values"=w1221) -> ()  [unwired: 1 in, 2 out]
                  }
                  frame #1 {
                    n895 = for {
                      N: 20 -> [_]
                      tunnel: w1226 -> [w1234]
                      tunnel: w1225 -> [w1229]
                      i -> [w1228]
                      n896 = Compound Arithmetic op=ADD(1.0 ("值"), w1229, w1228) -> (w1231:dbl)
                      n897 = Bundle(w1231, 0) -> (w1233:cluster{dbl, i32})  [unwired: 1 out]
                      n898 = property class="Tbl (严格)"(reference=w1234, "Active Cell"=w1233, "Cell BG Color"=u32 6618880) -> ()  [unwired: 1 in, 2 out]
                    }
                  }
                }
                n899 = Select(t=0, s=w1202, f=1) -> (s? t:f=w1203:i32)
                n900 = property on="项目信息" class="Tbl (严格)"("Disabled"=w1203) -> ()  [unwired: 2 in, 2 out]
                n901 = global read "功能码全局.vi" "主板项目信息5"() -> (w1210:bool[])
                n902 = global read "功能码全局.vi" "主板项目信息6"() -> (w1208:bool[])
                n903 = Index Array(array=w1210, index=2 ("索引")) -> (element=w1207:bool)
                n904 = Index Array(array=w1208, index=3 ("索引")) -> (element=w1206:bool)
                n905 = Not(x=w1216) -> (.not. x?=w1215:bool)
              }
              frame "电压起始值" {
                w1248 = 2
                w1250 = FALSE
                n906 = property on="从板个数" class="DigNum (严格)"("NumText.BGColor"=u32 13816530) -> ()  [unwired: 2 in, 2 out]
                n907 = property on="电池实际容量(A)" class="DigNum (严格)"("Disabled"=w1248) -> ()  [unwired: 2 in, 2 out]
                n908 = property on="使用者" class="DigNum (严格)"("Disabled"=w1248) -> ()  [unwired: 2 in, 2 out]
                n909 = property on="SOH(%)" class="DigNum (严格)"("Disabled"=w1248) -> ()  [unwired: 2 in, 2 out]
                n910 = property on="电池额定容量(A)" class="DigNum (严格)"("Disabled"=w1248) -> ()  [unwired: 2 in, 2 out]
                n911 = property on="SOC(%)" class="DigNum (严格)"("Disabled"=w1248) -> ()  [unwired: 2 in, 2 out]
                n912 = local read "从板个数"() -> (w1246:dbl)
                n913 = property on="系统时钟" class="Str"("Disabled"=w1248) -> ()  [unwired: 2 in, 2 out]
                n914 = property on="配置文件版本" class="Str"("Disabled"=w1248) -> ()  [unwired: 2 in, 2 out]
                n915 = property on="车架(牌)号" class="Str"("Disabled"=w1248) -> ()  [unwired: 2 in, 2 out]
                n916 = property on="产品编号" class="Str"("Disabled"=w1248) -> ()  [unwired: 2 in, 2 out]
                n917 = control-ref of="项目信息"() -> (w1247:refnum<vi>)
                n918 = stacked-sequence {
                  tunnel: w1247 -> [w1257 w1260 w1273]
                  tunnel: w1246 -> [w1256 w1259 w1272]
                  frame #0 {
                    n919 = Compound Arithmetic op=ADD(21.0 ("值"), w1256) -> (w1253:dbl)
                    n920 = Bundle(w1253, 0) -> (w1255:cluster{dbl, i32})  [unwired: 1 out]
                    n921 = property class="Tbl (严格)"(reference=w1257, "Index Values"=w1255) -> ()  [unwired: 1 in, 2 out]
                  }
                  frame #1 {
                    n922 = for {
                      N: 10 -> [_]
                      tunnel: w1260 -> [w1270]
                      tunnel: w1259 -> [w1265]
                      i -> [w1264]
                      n923 = Multiply(x=w1265, y=2.0) -> (x*y=w1262:dbl)
                      n924 = Compound Arithmetic op=ADD(21.0 ("值"), w1262, w1264) -> (w1267:dbl)
                      n925 = Bundle(w1267, 0) -> (w1269:cluster{dbl, i32})  [unwired: 1 out]
                      n926 = property class="Tbl (严格)"(reference=w1270, "Active Cell"=w1269, "Cell BG Color"=u32 16448250) -> ()  [unwired: 1 in, 2 out]
                    }
                  }
                  frame #2 {
                    n927 = Increment(x=w1272) -> (x+1=w1271:dbl)
                    n928 = for {
                      N: w1271 -> [_]
                      tunnel: w1273 -> [w1281]
                      tunnel: w1272 -> [w1276]
                      i -> [w1275]
                      n929 = Compound Arithmetic op=ADD(21.0 ("值"), w1276, w1275) -> (w1278:dbl)
                      n930 = Bundle(w1278, 0) -> (w1280:cluster{dbl, i32})  [unwired: 1 out]
                      n931 = property class="Tbl (严格)"(reference=w1281, "Active Cell"=w1280, "Cell BG Color"=u32 6618880) -> ()  [unwired: 1 in, 2 out]
                    }
                  }
                }
                n932 = Select(t=0, s=w1237, f=1) -> (s? t:f=w1236:i32)
                n933 = property on="项目信息" class="Tbl (严格)"("Disabled"=w1236) -> ()  [unwired: 2 in, 2 out]
                n934 = global read "功能码全局.vi" "主板项目信息5"() -> (w1244:bool[])
                n935 = global read "功能码全局.vi" "主板项目信息6"() -> (w1242:bool[])
                n936 = Index Array(array=w1244, index=3 ("索引")) -> (element=w1240:bool)
                n937 = Index Array(array=w1242, index=4 ("索引")) -> (element=w1241:bool)
                n938 = Not(x=w1250) -> (.not. x?=w1249:bool)
              }
              frame "温度个数" {
                w1295 = 2
                w1297 = FALSE
                n939 = property on="电池实际容量(A)" class="DigNum (严格)"("Disabled"=w1295) -> ()  [unwired: 2 in, 2 out]
                n940 = property on="使用者" class="DigNum (严格)"("Disabled"=w1295) -> ()  [unwired: 2 in, 2 out]
                n941 = property on="SOH(%)" class="DigNum (严格)"("Disabled"=w1295) -> ()  [unwired: 2 in, 2 out]
                n942 = property on="电池额定容量(A)" class="DigNum (严格)"("Disabled"=w1295) -> ()  [unwired: 2 in, 2 out]
                n943 = property on="SOC(%)" class="DigNum (严格)"("Disabled"=w1295) -> ()  [unwired: 2 in, 2 out]
                n944 = local read "从板个数"() -> (w1293:dbl)
                n945 = control-ref of="项目信息"() -> (w1294:refnum<vi>)
                n946 = stacked-sequence {
                  tunnel: w1294 -> [w1302 w1305 w1312]
                  tunnel: w1293 -> [w1299 w1304 w1311]
                  frame #0 {
                    n947 = Bundle("从板个数"=w1299, 0) -> (w1301:cluster{"从板个数":dbl, i32})  [unwired: 1 out]
                    n948 = property class="Tbl (严格)"(reference=w1302, "Index Values"=w1301) -> ()  [unwired: 1 in, 2 out]
                  }
                  frame #1 {
                    n949 = for {
                      N: 20 -> [_]
                      tunnel: w1305 -> [w1310]
                      tunnel: w1304 -> [_]
                      i -> [w1306]
                      n950 = Bundle(w1306, 0) -> (w1309:cluster{i32, i32})  [unwired: 1 out]
                      n951 = property class="Tbl (严格)"(reference=w1310, "Active Cell"=w1309, "Cell BG Color"=u32 16448250) -> ()  [unwired: 1 in, 2 out]
                    }
                  }
                  frame #2 {
                    n952 = for {
                      N: w1311 -> [_]
                      tunnel: w1312 -> [w1319]
                      tunnel: w1311 -> [w1313]
                      i -> [w1314]
                      n953 = Compound Arithmetic op=ADD(w1313, w1314) -> (w1316:dbl)
                      n954 = Bundle(w1316, 0) -> (w1318:cluster{dbl, i32})  [unwired: 1 out]
                      n955 = property class="Tbl (严格)"(reference=w1319, "Active Cell"=w1318, "Cell BG Color"=u32 6618880) -> ()  [unwired: 1 in, 2 out]
                    }
                  }
                }
                n956 = property on="系统时钟" class="Str"("Disabled"=w1295) -> ()  [unwired: 2 in, 2 out]
                n957 = property on="配置文件版本" class="Str"("Disabled"=w1295) -> ()  [unwired: 2 in, 2 out]
                n958 = property on="车架(牌)号" class="Str"("Disabled"=w1295) -> ()  [unwired: 2 in, 2 out]
                n959 = property on="产品编号" class="Str"("Disabled"=w1295) -> ()  [unwired: 2 in, 2 out]
